vi "read_coef_init.vi"(8 "error in (no error)":errorcluster, 11 "Perceptron in":refnum<class "Perceptron.lvclass">) -> (0 "error out":errorcluster, 2 "coef_init":dbl[][](array[numeric]), 3 "Perceptron out":refnum<class "Perceptron.lvclass">)   [LabVIEW 2020, in "Perceptron.lvclass"]
uses:
  Perceptron.lvclass
  Perceptron.lvclass/Perceptron.ctl
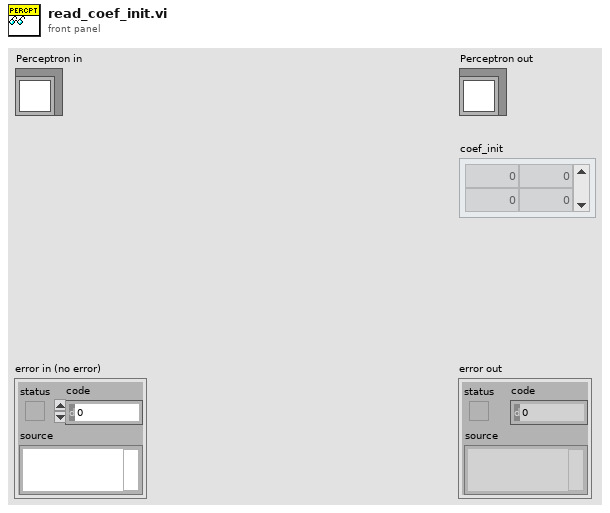
[diagram p1: front panel]
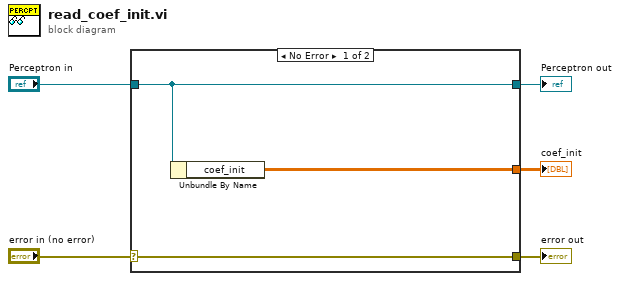
[diagram p0: block diagram]
diagram:
  n1 = case shown="No Error" "error in (no error)" {
    selector: "error in (no error)" -> [w8 w9]
    tunnel: [w8 w9] -> w4
    tunnel: [w7 w10] -> w2
    tunnel: "Perceptron in" -> [w7 w10]
    tunnel: [w6 _] -> w1
    frame No Error {
      n2 = Unbundle By Name(w7) -> ("coef_init"=w6:dbl[][])
    }
    frame Error {
    }
  }
  "error out" <- w4
  "Perceptron out" <- w2
  "coef_init" <- w1
